vi "Register for Actor Core Events.vi"(8 "error in (no error)":errorcluster, 9 "Controls to Exclude":refnum<vi>[](array[refnum]), 10 "VI Refnum (Calling VI)":refnum<vi>, 11 "Actor Enqueuer":refnum<class "Message Enqueuer.lvclass">) -> (0 "error out":errorcluster, 3 "ActorAutoRegistration Out":refnum<class "ActorAutoRegistration.lvclass">)   [LabVIEW 2015, in "ActorAutoRegistration.lvlib" / "ActorAutoRegistration.lvclass"]
uses:
  ActorAutoRegistration.lvclass
  <vilib>/ActorFramework/Message Enqueuer/Message Enqueuer.lvclass
  ActorAutoRegistration.lvclass/ActorAutoRegistration.ctl
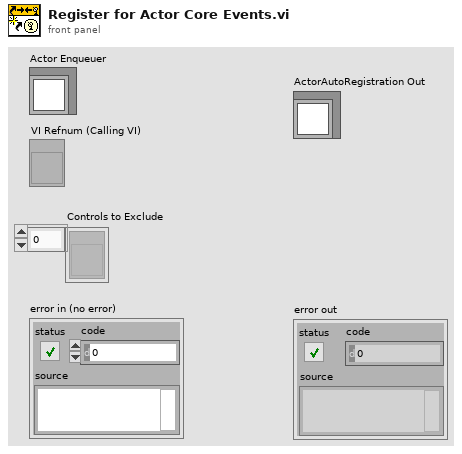
[diagram p1: front panel]
types:
  T1 = enum32{"Invalid", "Standard", "Closed", "Hidden", "Minimized", "Maximized"}
  T2 = typedef "AutoRegistration.lvlib/AutoRegistration.lvclass/Registration References.ctl" = cluster{"Switching Boolean":refnum<vi>[], "Latching Boolean":refnum<vi>[], "I8":refnum<vi>[], "I16":refnum<vi>[], "I32":refnum<vi>[], "I64":refnum<vi>[], "U8":refnum<vi>[], "U16":refnum<vi>[], "U32":refnum<vi>[], "U64":refnum<vi>[], "SGL":refnum<vi>[], "DBL":refnum<vi>[], "EXT":refnum<vi>[], "FXP":refnum<vi>[], "String":refnum<vi>[], "Path":refnum<vi>[], "Timestamp":refnum<vi>[], "Other Controls":refnum<vi>[]}
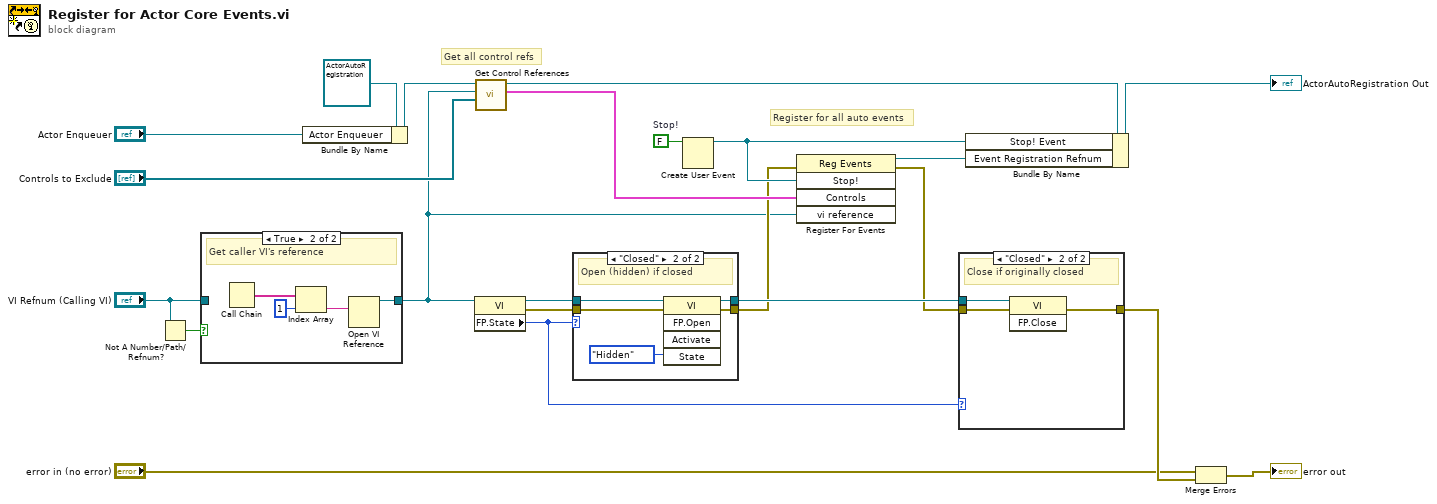
[diagram p0: block diagram]
diagram:
  w21 = FALSE  # Stop!
  # "Get all control refs"
  # "Register for all auto events"
  n1 = Not A Number/Path/Refnum?(number/path/refnum="VI Refnum (Calling VI)") -> (NaN/Path/Refnum?=w3:bool)
  n2 = case shown="True" w3 {
    tunnel: [w23 w24] -> w2
    tunnel: "VI Refnum (Calling VI)" -> [w23 _]
    frame False {
      # "Reference wired to input"
    }
    frame True {
      # "Get caller VI's reference"
      n3 = Call Chain() -> (call chain=w27:string[])
      n4 = Index Array(array=w27, index=1) -> (element=w25:string)
      n5 = Open VI Reference(vi path=w25) -> (vi reference=w24:refnum<vi>)  [unwired: 5 in, 1 out]
    }
  }
  n6 = Bundle By Name(cluster=refnum<class "ActorAutoRegistration.lvclass"> refnum ("AbstractAutoRegistration in"), "Actor Enqueuer"="Actor Enqueuer") -> (w4:refnum<class "ActorAutoRegistration.lvclass">)
  n7 = property on="Property Node" class="VI"(reference=w2) -> (reference out=w19:refnum<vi>, error out=w16:errorcluster, "FP.State"=w17:T1)  [unwired: 1 in]
  n8 = call-dynamic "Get Control References.vi"("Controls to Exclude"="Controls to Exclude", "VI Refnum"=w2, "AutoRegistration In"=w4) -> ("Controls"=w22:T2, "AutoRegistration Out"=w20:refnum<class "ActorAutoRegistration.lvclass">)  [unwired: 6 in, 1 out]
  n9 = case shown="\"Closed\"" w17 {
    tunnel: w19 -> [w29 w33]
    tunnel: [w28 w32] -> w8
    tunnel: [w29 w31] -> w18
    tunnel: w16 -> [w28 w30]
    frame Default {
      # "Do nothing"
    }
    frame "Closed" {
      # "Open (hidden) if closed"
      n10 = invoke on="Invoke Node" class="VI" method="FP.Open"(reference=w33, error in=w30, "State"=T1."Hidden") -> (reference out=w31:refnum<vi>, error out=w32:errorcluster)  [unwired: 2 in, 3 out]
    }
  }
  n11 = Create User Event(user event datatype=w21) -> (user event=w9:refnum<user-event>)  [unwired: 1 in, 1 out]
  n12 = register-events(error in=w8, w9, w22, w2) -> (reference out=w11:refnum<event-registration>, error out=w15:errorcluster)  [unwired: 1 in]
  n13 = case shown="\"Closed\"" w17 {
    tunnel: w18 -> [_ w37]
    tunnel: w15 -> [_ w35]
    tunnel: [_ w36] -> w10
    frame Default {
      # "Do nothing"
    }
    frame "Closed" {
      # "Close if originally closed"
      n14 = invoke on="Invoke Node" class="VI" method="FP.Close"(reference=w37, error in=w35) -> (error out=w36:errorcluster)  [unwired: 1 in, 2 out]
    }
  }
  n15 = Bundle By Name(cluster=w20, "Stop! Event"=w9, "Event Registration Refnum"=w11) -> (→"ActorAutoRegistration Out":refnum<class "ActorAutoRegistration.lvclass">)
  n16 = Merge Errors("error in (no error)", w10) -> (→"error out":errorcluster)
